vi "csm_lumikki_instron_status_poller_backup.vi"() -> ()   [LabVIEW 2009]
uses:
  Documents and Settings/All Users/Documents/Instron/FastTrack3/Common/MultiAxis/Arbitrator Interface/MX Arbitrator Globals.vi
panel:
  out "Boolean array":bool[](array[boolean])
  out "Success 4":bool
  out "Bytes Read":i32
  out "Success 3":bool
  out "Rebuilt Status String 2":string
  out "Rebuilt Status String":string
  out "Success 2":bool
  out "Success":bool
  out "GPIB Group":i32
  out "Group Name":string
  out "error out":errorcluster
  out "Error in obtaining\ngroup ID from user":bool
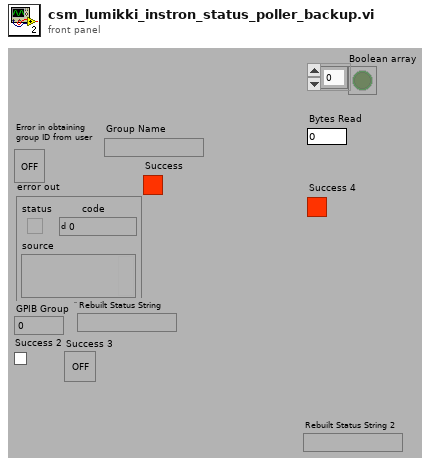
[diagram p1: front panel]
types:
  T1 = cluster{"Device ID":i32, "Device Name":string, "Device Type":i32}[]
  T2 = cluster{"Device ID":i32, "GPIB Group Number":i32, "Device Type":i32, "Device Name":string}[]
  T3 = cluster{"MX Array of GPIB device Information[0]":cluster{"Device ID":i32, "GPIB Group Number":i32, "Device Type":i32, "Device Name":string}, "MX Array of GPIB device Information[1]":cluster{"Device ID":i32, "GPIB Group Number":i32, "Device Type":i32, "Device Name":string}, "MX Array of GPIB device Information[2]":cluster{"Device ID":i32, "GPIB Group Number":i32, "Device Type":i32, "Device Name":string}, "MX Array of GPIB device Information[3]":cluster{"Device ID":i32, "GPIB Group Number":i32, "Device Type":i32, "Device Name":string}, "MX Array of GPIB device Information[4]":cluster{"Device ID":i32, "GPIB Group Number":i32, "Device Type":i32, "Device Name":string}, "MX Array of GPIB device Information[5]":cluster{"Device ID":i32, "GPIB Group Number":i32, "Device Type":i32, "Device Name":string}, "MX Array of GPIB device Information[6]":cluster{"Device ID":i32, "GPIB Group Number":i32, "Device Type":i32, "Device Name":string}, "MX Array of GPIB device Information[7]":cluster{"Device ID":i32, "GPIB Group Number":i32, "Device Type":i32, "Device Name":string}, "MX Array of GPIB device Information[8]":cluster{"Device ID":i32, "GPIB Group Number":i32, "Device Type":i32, "Device Name":string}}
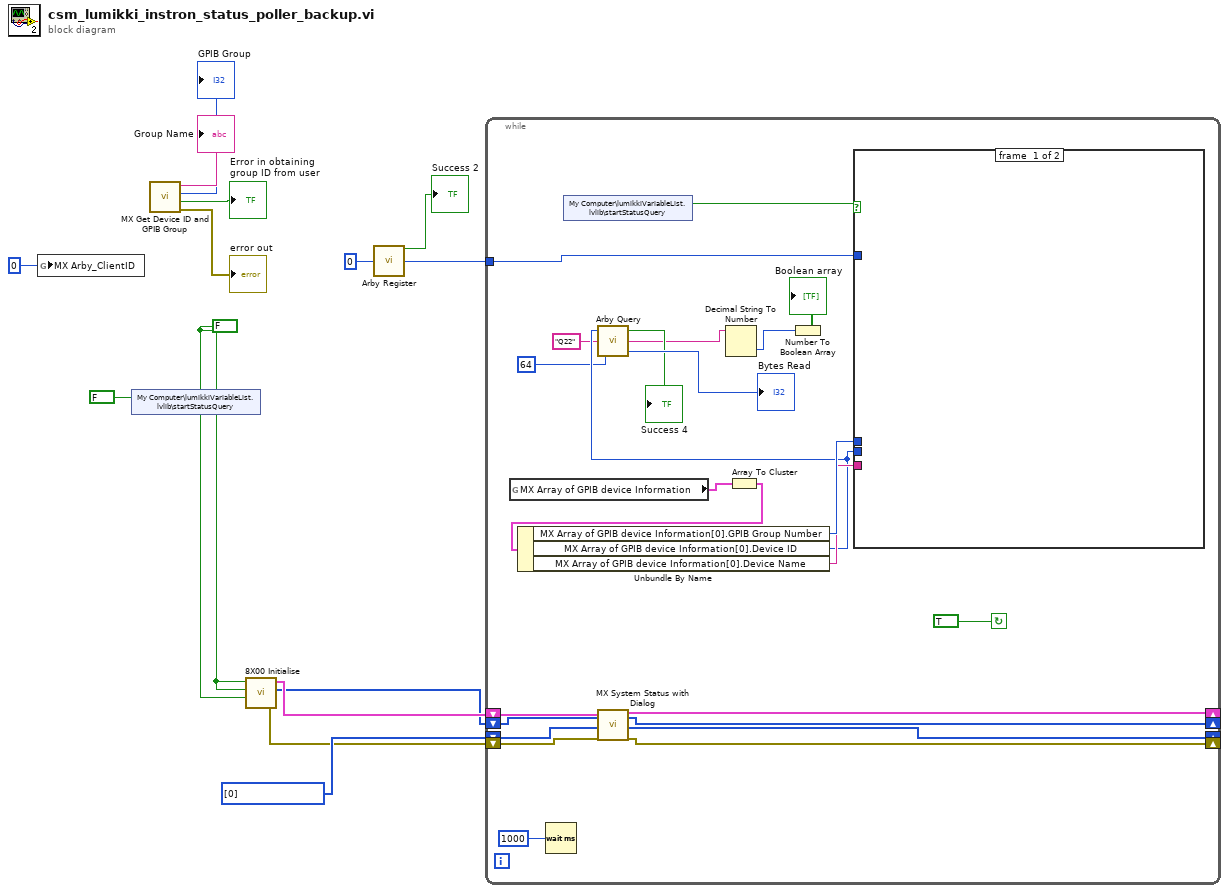
[diagram p0: block diagram]
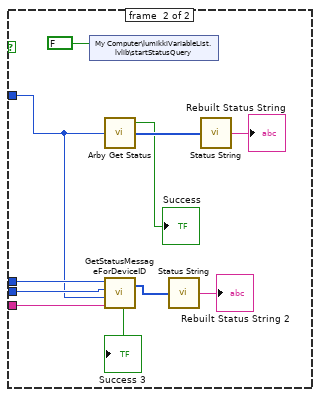
[diagram p2: hidden frame]
diagram:
  w2 = u16[] [0] items=["Channel 1", "Channel 2", "Channel 3", "Channel 4"] ("Channels In")
  w14 = FALSE ("Create Console? (T)")
  n1 = global write "MX Arbitrator Globals.vi" "MX Arby_ClientID"(0 ("MX Arby_ClientID")) -> ()
  n2 = shared-variable "My Computer\\lumikkiVariableList.lvlib\\startStatusQuery"(FALSE ("startStatusQuery")) -> ()  [unwired: 1 in, 1 out]
  n3 = call "MX Get Device ID and GPIB Group.vi"() -> ("Group Name"=→"Group Name":string, "GPIB Group"=→"GPIB Group":i32, "Error in obtaining\ngroup ID from user"=→"Error in obtaining\ngroup ID from user":bool, "error out"=→"error out":errorcluster)  [unwired: 3 in]
  n4 = call "8X00 Initialise.vi"("Reset?"=w14, "Create DVM? (T)"=w14, "Create Console? (T)"=w14) -> ("error out"=w1:errorcluster, "Axis Selector"=w3:i32[], "Axis Information"=w4:T1)  [unwired: 1 in, 1 out]
  n5 = call "Arby Register.vi"("Mask"=0) -> ("Success"=→"Success 2":bool, "Arby_ClientID"=w7:i32)  [unwired: 12 in, 1 out]
  n6 = while {
    tunnel: w7 -> [w36]
    shift-right: [w31] -> _
    shift-left: w4 -> [w15]
    shift-right: [w30] -> _
    shift-left: w3 -> [w27]
    shift-right: [w29] -> _
    shift-left: w2 -> [w26]
    shift-right: [w28] -> _
    shift-left: w1 -> [w25]
    stop <- TRUE continue-if-true
    n7 = global read "MX Arbitrator Globals.vi" "MX Array of GPIB device Information"() -> (w35:T2)
    n8 = Wait (ms)(milliseconds to wait=u32 1000) -> ()  [unwired: 1 out]
    n9 = shared-variable "My Computer\\lumikkiVariableList.lvlib\\startStatusQuery"() -> (w37:bool)  [unwired: 1 in, 1 out]
    n10 = call "MX System Status with Dialog.vi"("Axis Information In"=w15, "Axis Selector In"=w27, "Channels In"=w26, "Error In"=w25) -> ("Axis Information Out"=w31:T1, "Axis Selector Out"=w30:i32[], "Channels Out"=w29:u16[], "Error Out"=w28:errorcluster)  [unwired: 10 in, 2 out]
    n11 = Array To Cluster(array=w35) -> (cluster=w34:T3)
    n12 = Unbundle By Name(w34) -> ("MX Array of GPIB device Information[0].GPIB Group Number"=w33:i32, "MX Array of GPIB device Information[0].Device ID"=w24:i32, "MX Array of GPIB device Information[0].Device Name"=w32:string)
    n13 = call "Arby Query.vi"("Reply size"=64, "Query"="Q22", "Device"=w24) -> ("Bytes Read"=→"Bytes Read":i32, "Reply"=w18:string, "Success"=→"Success 4":bool)
    n14 = Decimal String To Number(string=w18) -> (number=w17:i32)  [unwired: 2 in, 1 out]
    n15 = Number To Boolean Array(number=w17) -> (Boolean array=→"Boolean array":bool[])
    n16 = case shown="True" w37 {
      tunnel: w36 -> [_ w43]
      tunnel: w33 -> [_ w45]
      tunnel: w24 -> [_ w44]
      tunnel: w32 -> [_ w42]
      frame #0 {
      }
      frame #1 {
        n17 = shared-variable "My Computer\\lumikkiVariableList.lvlib\\startStatusQuery"(FALSE ("startRamp")) -> ()  [unwired: 1 in, 1 out]
        n18 = call "Arby Get Status.vi"("Arby_ClientID"=w43) -> ("Success"=→"Success":bool, "Status"=w48:i32[])  [unwired: 1 out]
        n19 = call "GetStatusMessageForDeviceID.vi"("Device Name"=w42, "Arbitrator\nClient ID"=w43, "DeviceID"=w44, "Arbitrator GPIB Group"=w45) -> ("Success"=→"Success 3":bool, "Status Output"=w40:i32[])
        n20 = call "Status String.vi"("Status Input"=w40) -> ("Rebuilt Status String"=→"Rebuilt Status String 2":string)
        n21 = call "Status String.vi"("Status Input"=w48) -> ("Rebuilt Status String"=→"Rebuilt Status String":string)
      }
    }
  }
